vi "Remove Team by ID.vi"(8 "error in (no error)":errorcluster, 10 "Team ID":T1 format="%.0x", 11 "Game in":refnum<class "Game.lvclass">) -> (0 "error out":errorcluster, 3 "Game out":refnum<class "Game.lvclass">)   [LabVIEW 2020, in "SquareBattle.lvlib" / "Game.lvclass"]
uses:
  Game.lvclass
  Team ID.ctl
  Game.lvclass/Game.ctl
  SquareBattle.lvlib
  Team/Team.lvclass
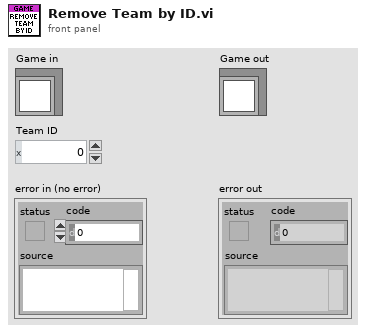
[diagram p1: front panel]
types:
  T1 = typedef "SquareBattle.lvlib/Team ID.ctl" = u32
  T2 = typedef "SquareBattle.lvlib/Position.ctl" = cluster{"Row":i32, "Col":i32}
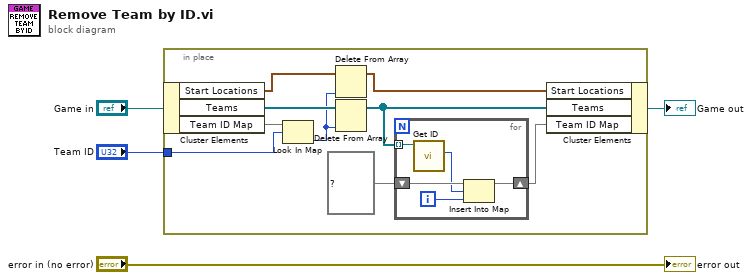
[diagram p0: block diagram]
diagram:
  n1 = in-place {
    in-place-border: "Team ID" -> [w11]
    n2 = in-place-cluster #1("Game in") -> ("Start Locations"=w9:T2[], "Teams"=w13:refnum<class "Team.lvclass">[], "Team ID Map"=w12:map{T1, i32})
    n3 = Look In Map(map=w12, key=w11) -> (value=w10:i32)  [unwired: 1 in, 1 out]
    n4 = Delete From Array(array=w9, index=w10) -> (array with subset deleted=w8:T2[])  [unwired: 1 in, 1 out]
    n5 = Delete From Array(array=w13, index=w10) -> (array with subset deleted=w7:refnum<class "Team.lvclass">[])  [unwired: 1 in, 1 out]
    n6 = for {
      tunnel: w7 -> [w17] mode=indexing
      shift-right: [w14] -> w5
      shift-left: map{T1, i32} {} ("Team ID Map") -> [w18]
      i -> [w15]
      n7 = call "Get ID.vi"("Team in"=w17) -> ("Team ID"=w16:T1)  [unwired: 10 in]
      n8 = Insert Into Map(map in=w18, key=w16, value=w15) -> (map out=w14:map{T1, i32})  [unwired: 2 out]
    }
    n9 = in-place-cluster #1("Start Locations"=w8, "Teams"=w7, "Team ID Map"=w5) -> (→"Game out":refnum<class "Game.lvclass">)
  }
  "error out" <- "error in (no error)"
